vi "Dynamic Test.vi"(5 "Mechanical Zero":dbl, 9 "read buffer":string) -> (4 "Elbow Angle (deg)":dbl, 6 "Goniometer\nAngle Raw":dynamicdata(graph), 8 "Dynamic LF":dbl, 10 "Dynamic Load Force":dynamicdata(graph), 14 "Grip Force":dynamicdata(graph), 15 "GF":dbl)   [LabVIEW 2018]
doc: "VI for GF and LF conversion."
panel:
  out "Static LF":dbl
  # "\"Throw away\" data"
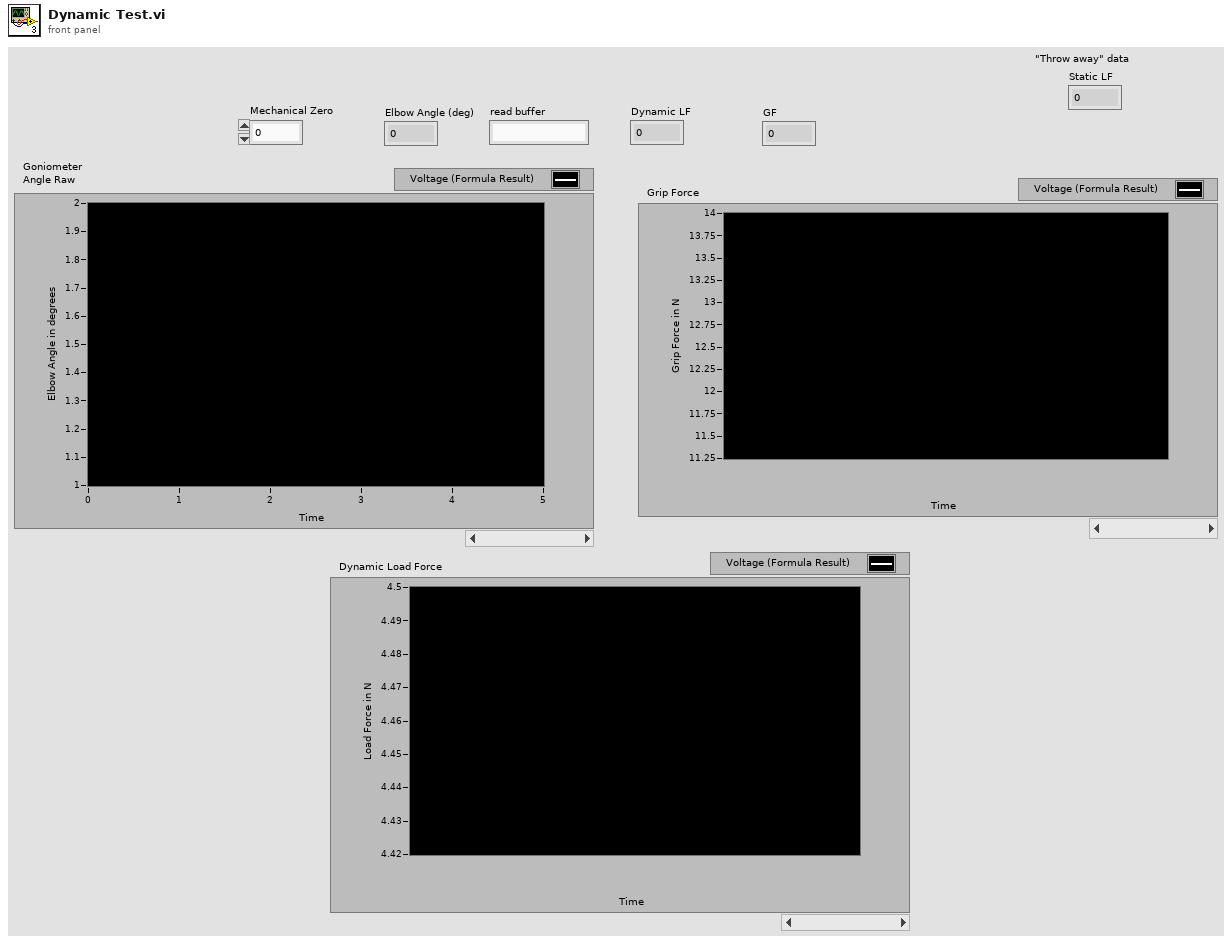
[diagram p1: front panel]
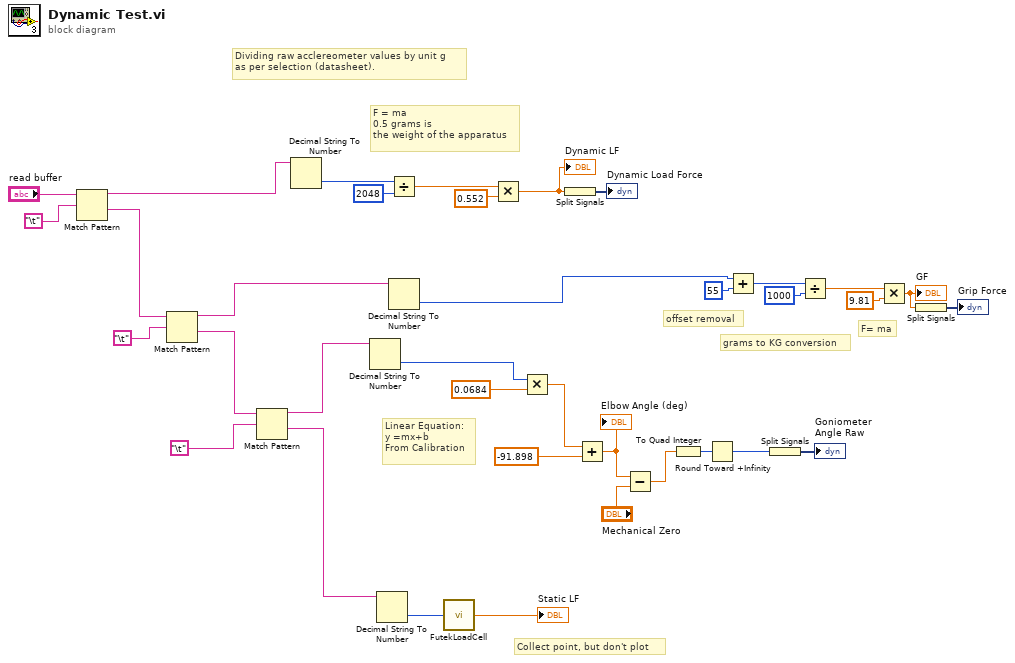
[diagram p0: block diagram]
diagram:
  # "F = ma\n0.5 grams is \nthe weight of the apparatus"
  # "Dividing raw acclereometer values by unit g\nas per selection (datasheet)."
  # "Collect point, but don't plot"
  # "F= ma"
  # "offset removal"
  # "grams to KG conversion"
  # "Linear Equation:\ny =mx+b\nFrom Calibration"
  n1 = Match Pattern(string="read buffer", regular expression="\t") -> (before substring=w36:string, after substring=w32:string)  [unwired: 1 in, 2 out]
  n2 = Match Pattern(string=w32, regular expression="\t") -> (before substring=w31:string, after substring=w20:string)  [unwired: 1 in, 2 out]
  n3 = Match Pattern(string=w20, regular expression="\t") -> (before substring=w19:string, after substring=w18:string)  [unwired: 1 in, 2 out]
  n4 = Decimal String To Number(string=w36) -> (number=w4:i32)  [unwired: 2 in, 1 out]
  n5 = Decimal String To Number(string=w19) -> (number=w26:i32)  [unwired: 2 in, 1 out]
  n6 = Decimal String To Number(string=w18) -> (number=w2:i32)  [unwired: 2 in, 1 out]
  n7 = Divide(x=w4, y=2048) -> (x/y=w8:dbl)
  n8 = Decimal String To Number(string=w31) -> (number=w9:i32)  [unwired: 2 in, 1 out]
  n9 = call "FutekLoadCell.vi"("Futek Sensor Reading"=w2) -> ("Futek Force"=→"Static LF":dbl)
  n10 = Multiply(x=w8, y=0.552) -> (x*y=w7:dbl)
  "Dynamic LF" <- w7
  n11 = Multiply(x=w26, y=0.0684 ("x")) -> (x*y=w29:dbl)
  n12 = Split Signals(w7) -> (→"Dynamic Load Force":dynamicdata)  [unwired: 1 in]
  n13 = Add(x=w29, y=-91.898 ("x")) -> (x+y=w24:dbl)
  "Elbow Angle (deg)" <- w24
  n14 = Subtract(x=w24, y="Mechanical Zero") -> (x-y=w25:dbl)
  n15 = To Quad Integer(1:w25) -> (0:w22:i64)
  n16 = Round Toward +Infinity(x=w22) -> (ceil(x): smallest int >= x=w21:i64)
  n17 = Add(x=w9, y=55) -> (x+y=w15:i32)
  n18 = Split Signals(w21) -> (→"Goniometer\nAngle Raw":dynamicdata)  [unwired: 1 in]
  n19 = Divide(x=w15, y=1000) -> (x/y=w12:dbl)
  n20 = Multiply(x=w12, y=9.81) -> (x*y=w16:dbl)
  "GF" <- w16
  n21 = Split Signals(w16) -> (→"Grip Force":dynamicdata)  [unwired: 1 in]
